vi "Dodawanie punktu na podstawie odległości od robota w kierunku xy.vi"(7 "Parametry odwzorowania Ziemi":cluster{"a":dbl, "b":dbl}={"a"=6378137.0, "b"=6356752.3142} {"b" format="%#.12g"; "a" format="%#.12g"}, 9 "Zaznaczony punkt":T2, 10 "Początkowe UTM":T1={"E_coord[m]"=393271.81, "N_coord[m]"=5734673.27, "Strefa"=""}, 11 "Lista współrzędnych":string[][](array[string])) -> (3 "output array":string[][](array[string]))   [LabVIEW 2012, in "Biblioteka moduł map v3.lvlib" / "Obsługa listy współrzędnych.lvlib"]
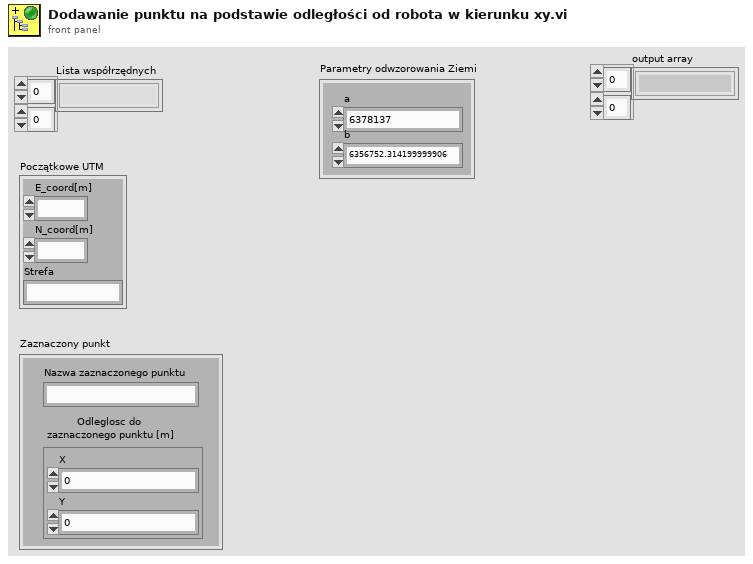
[diagram p1: front panel]
types:
  T1 = cluster{"E_coord[m]":ext, "N_coord[m]":ext, "Strefa":string}
  T2 = cluster{"Nazwa zaznaczonego punktu":string, "Odleglosc do\n zaznaczonego punktu [m]":cluster{"X":dbl, "Y":dbl}}
  T3 = cluster{"fi - szerokość geograficzna":ext, "lambda - długość geograficzna":ext}
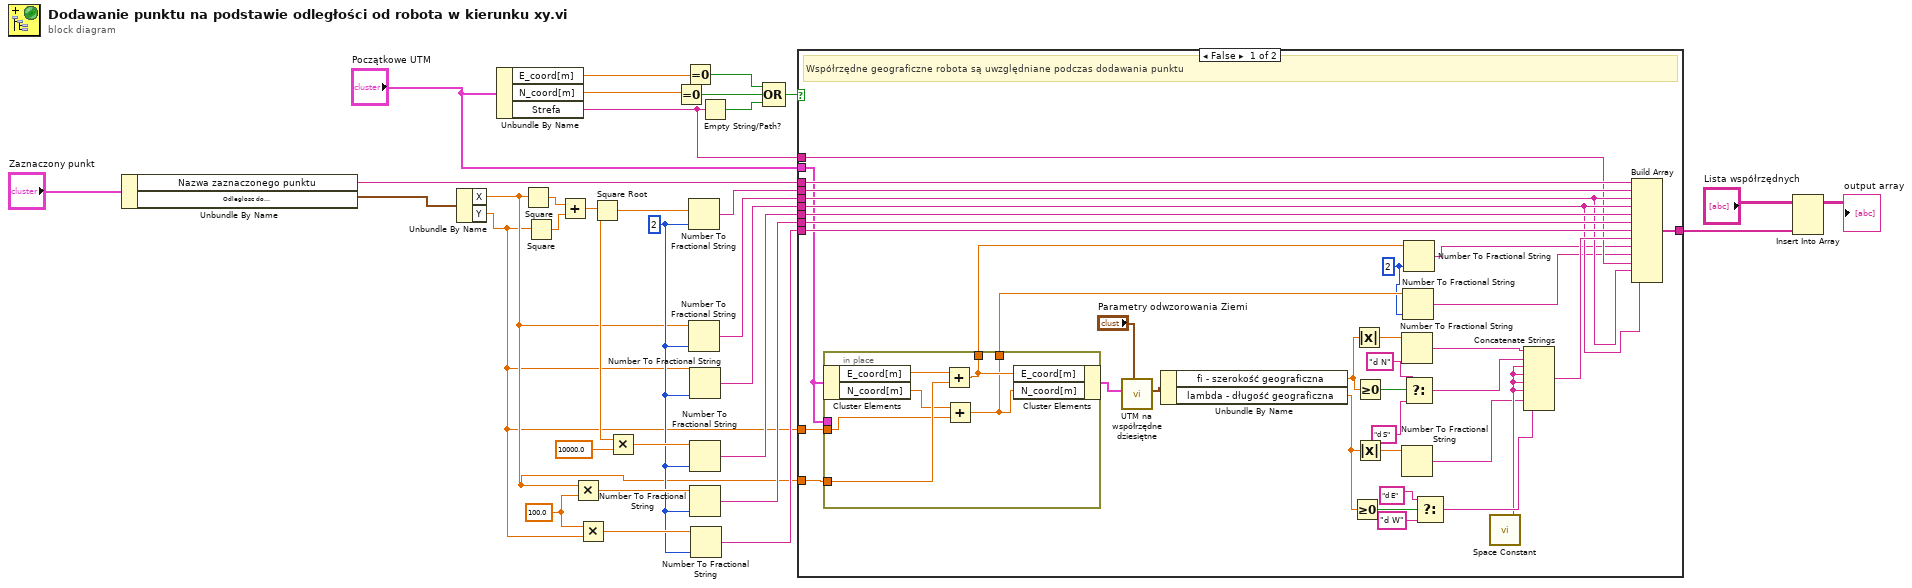
[diagram p0: block diagram]
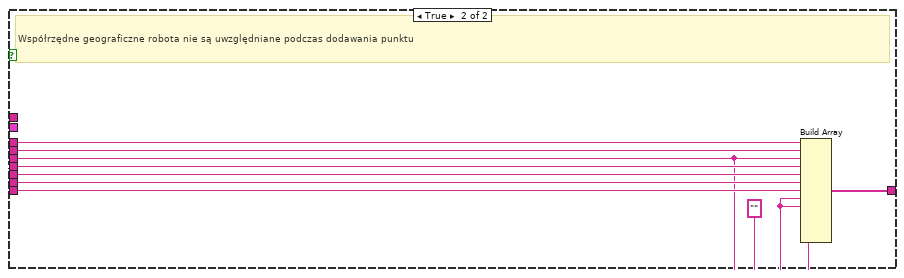
[diagram p2: hidden frame]
diagram:
  w18 = i16 2 ("precision (6)")
  w15 = 100.0 ("y")
  n1 = Unbundle By Name("Zaznaczony punkt") -> ("Nazwa zaznaczonego punktu"=w25:string, "Odleglosc do\n zaznaczonego punktu [m]"=w26:cluster{"X":dbl, "Y":dbl})
  n2 = Unbundle By Name(w26) -> ("X"=w3:dbl, "Y"=w2:dbl)
  n3 = Unbundle By Name("Początkowe UTM") -> ("E_coord[m]"=w6:ext, "N_coord[m]"=w5:ext, "Strefa"=w4:string)
  n4 = Square(x=w3) -> (x^2=w8:dbl)
  n5 = Square(x=w2) -> (x^2=w9:dbl)
  n6 = Add(x=w8, y=w9) -> (x+y=w10:dbl)
  n7 = Multiply(x=w3, y=w15) -> (x*y=w22:dbl)
  n8 = Multiply(x=w15, y=w2) -> (x*y=w23:dbl)
  n9 = Square Root(x=w10) -> (sqrt(x)=w17:dbl)
  n10 = Multiply(x=w17, y=10000.0) -> (x*y=w21:dbl)
  n11 = Equal To 0?(x=w5) -> (x = 0?=w28:bool)
  n12 = Equal To 0?(x=w6) -> (x = 0?=w29:bool)
  n13 = Number To Fractional String(number=w17, precision (6)=w18) -> (F-format string=w11:string)  [unwired: 2 in]
  n14 = Number To Fractional String(number=w3, precision (6)=w18) -> (F-format string=w19:string)  [unwired: 2 in]
  n15 = Number To Fractional String(number=w2, precision (6)=w18) -> (F-format string=w20:string)  [unwired: 2 in]
  n16 = Number To Fractional String(number=w21, precision (6)=w18) -> (F-format string=w12:string)  [unwired: 2 in]
  n17 = Number To Fractional String(number=w22, precision (6)=w18) -> (F-format string=w13:string)  [unwired: 2 in]
  n18 = Number To Fractional String(number=w23, precision (6)=w18) -> (F-format string=w14:string)  [unwired: 2 in]
  n19 = Empty String/Path?(string/path=w4) -> (empty?=w27:bool)
  n20 = Compound Arithmetic op=OR(w29, w28, w27) -> (w7:bool)
  n21 = case shown="False" w7 {
    tunnel: w25 -> [w68 w83]
    tunnel: [w63 w82] -> w24
    tunnel: w20 -> [w44 w81]
    tunnel: w19 -> [w43 w75]
    tunnel: w14 -> [w64 w79]
    tunnel: w13 -> [w65 w78]
    tunnel: w12 -> [w66 w77]
    tunnel: w11 -> [w67 w76]
    tunnel: "Początkowe UTM" -> [w34 _]
    tunnel: w4 -> [w42 _]
    tunnel: w3 -> [w41 _]
    tunnel: w2 -> [w40 _]
    frame False {
      w37 = i16 2 ("precision (6)")
      # "Współrzędne geograficzne robota są uwzględniane podczas dodawania punktu"
      n22 = in-place {
        in-place-border: w34 -> [_]
        in-place-border: w41 -> [w74]
        in-place-border: w40 -> [w69]
        in-place-border: [w71] -> w39
        in-place-border: [w70] -> w38
        n23 = in-place-cluster #1(w34) -> ("E_coord[m]"=w73:ext, "N_coord[m]"=w72:ext)
        n24 = Add(x=w73, y=w74) -> (x+y=w71:ext)
        n25 = Add(x=w72, y=w69) -> (x+y=w70:ext)
        n26 = in-place-cluster #1("E_coord[m]"=w71, "N_coord[m]"=w70) -> (w33:T1)
      }
      n27 = call "UTM na współrzędne dziesiętne.vi"("Parametry Ziemi"="Parametry odwzorowania Ziemi", "UTM"=w33) -> ("Położenie we współrzędnych geograficznych"=w47:T3)  [unwired: 8 in]
      n28 = Unbundle By Name(w47) -> ("fi - szerokość geograficzna"=w46:ext, "lambda - długość geograficzna"=w45:ext)
      n29 = Greater Or Equal To 0?(x=w45) -> (x >= 0?=w52:bool)
      n30 = Absolute Value(x=w46) -> (abs(x)=w54:ext)
      n31 = Greater Or Equal To 0?(x=w46) -> (x >= 0?=w53:bool)
      n32 = Absolute Value(x=w45) -> (abs(x)=w55:ext)
      n33 = Number To Fractional String(number=w54) -> (F-format string=w49:string)  [unwired: 3 in]
      n34 = Number To Fractional String(number=w55) -> (F-format string=w50:string)  [unwired: 3 in]
      n35 = Number To Fractional String(number=w38, precision (6)=w37) -> (F-format string=w35:string)  [unwired: 2 in]
      n36 = Number To Fractional String(number=w39, precision (6)=w37) -> (F-format string=w36:string)  [unwired: 2 in]
      n37 = Select(t="d N", s=w53, f="d S") -> (s? t:f=w60:string)
      n38 = Select(t="d E", s=w52, f="d W") -> (s? t:f=w62:string)
      n39 = call <vilib>:"Space Constant.vi"() -> ("String"=w61:string)
      n40 = Concatenate Strings(w49, w60, w61, w61, w61, w61, w50, w62) -> (w51:string)
      n41 = Build Array(w68, w67, w43, w44, w66, w65, w64, w51, w36, w35, w42, w43, w44) -> (w63:string[])
    }
    frame True {
      w80 = "" ("element")
      # "Współrzędne geograficzne robota nie są uwzględniane podczas dodawania punktu"
      n42 = Build Array(w83, w76, w75, w81, w77, w78, w79, w80, w80, w80, w80, w75, w81) -> (w82:string[])
    }
  }
  n43 = Insert Into Array(array="Lista współrzędnych", new element=w24) -> (→"output array":string[][])  [unwired: 2 in]
